vi "Humidification.vi"(10 "Humidifier":string="med", 11 "Controller in":refnum<class "Controller.lvclass">) -> ()   [LabVIEW 2018, in "Controller.lvlib" / "Controller.lvclass"]
doc: "This VI handles the humidifier loop."
uses:
  Controller.lvclass
  <vilib>/ActorFramework/Message Enqueuer/Message Enqueuer.lvclass
  Controls/eMap.ctl
  Devices/Vaisala Probe/Data/Vaisala Data.lvclass
  reusable/Session APIs/Session Log/System Log.lvclass
  <vilib>/ActorFramework/Actor/Actor.lvclass
  <vilib>/Platform/TimedLoop/XDataNode/XDataNode.xnode
  <vilib>/Platform/TimedLoop/XDataNode/nitl_modes.ctl
  <vilib>/Platform/TimedLoop/XDataNode/XDNodeRunTimeDep.lvlib
  <vilib>/Platform/TimedLoop/XDataNode/wakeup.ctl
  <vilib>/Platform/TimedLoop/XDataNode/timing_clust.ctl
  Devices/Meerstetter TEC/Data/mTEC Data.lvclass
  Devices/Alicat/Session Based/Data/Alicat Data.lvclass
  Update Controller Data MSG.lvclass
  Messages/Update Device Setpoint MSG/Update Device Setpoint.lvclass
  Data/humidity/humData.lvclass
  C:/Users/Labview/Documents/exscalabar_server/reusable/Data/Data.lvclass
  C:/Users/Labview/Documents/exscalabar_server/reusable/DAQ Device/Device/Generic Data Update Data MSG/Generic Update Data Message.lvclass
  C:/Program Files (x86)/National Instruments/LabVIEW 2018/vi.lib/ActorFramework/Message/Message.lvclass
  C:/Users/Labview/Documents/exscalabar_server/SuperActor/SuperActor.lvclass
  C:/Program Files (x86)/National Instruments/LabVIEW 2018/vi.lib/ActorFramework/Actor/Actor.lvclass
panel:
  out "TdReq":dbl
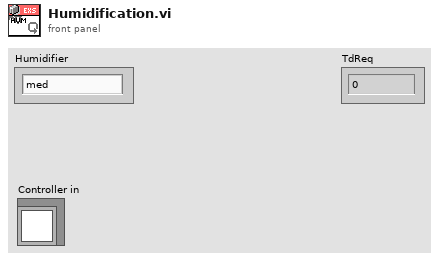
[diagram p1: front panel]
types:
  T1 = typedef "Session - Root.lvclass/Session Handle.ctl" = refnum<data-value>
  T2 = typedef "XDNodeRunTimeDep.lvlib/timing_clust.ctl" = cluster{"Expected End [f-1]":u64, "Actual End [f-1]":u64, "Finished Late? [f-1]":bool, "Expected End [i-1]":u64, "Actual End [i-1]":u64, "Finished Late? [i-1]":bool, "Expected Start [i]":u64, "Actual Start [i]":u64, "Expected Start [f]":u64, "Actual Start [f]":u64, "Source Name":string, "Structure Name":string, "Period":i64, "Deadline":i64, "Offset":i64, "Start":i64, "Priority":i32, "Timeout":i32, "Mode":T3, "Wakeup Reason":T4, "Error":errorcluster, "Source Type":string, "Secondary Source Type":string, "Global End Time":u64, "Global Start Time":u64, "Frame Duration":u64, "Iteration Duration":u64, "Assigned CPU":i32, "I/O Scan Engine Mode":u32}
  T3 = typedef "XDNodeRunTimeDep.lvlib/nitl_modes.ctl" = enum32{"No Change", "Process missed periods, maintain original phase", "Discard missed periods, maintain original phase", "Process missed periods, ignore original phase", "Discard missed periods, ignore original phase"}
  T4 = typedef "XDNodeRunTimeDep.lvlib/wakeup.ctl" = enum32{"Normal", "Aborted", "Asynchronous wakeup", "Timing source error", "Timed loop error", "Timeout"}
  T5 = typedef "Controller.lvlib/Controller.lvclass/eMap.ctl" = cluster{"Enqueuer":refnum<class "Message Enqueuer.lvclass">, "Active":bool}
  T6 = cluster{"Heff":dbl, "Leff":dbl, "dt":dbl, "smooth":dbl, "RHsp":dbl}
  T7 = cluster{"P":sgl, "T":sgl, "Q":sgl, "Qsp":sgl, "Q0":sgl}
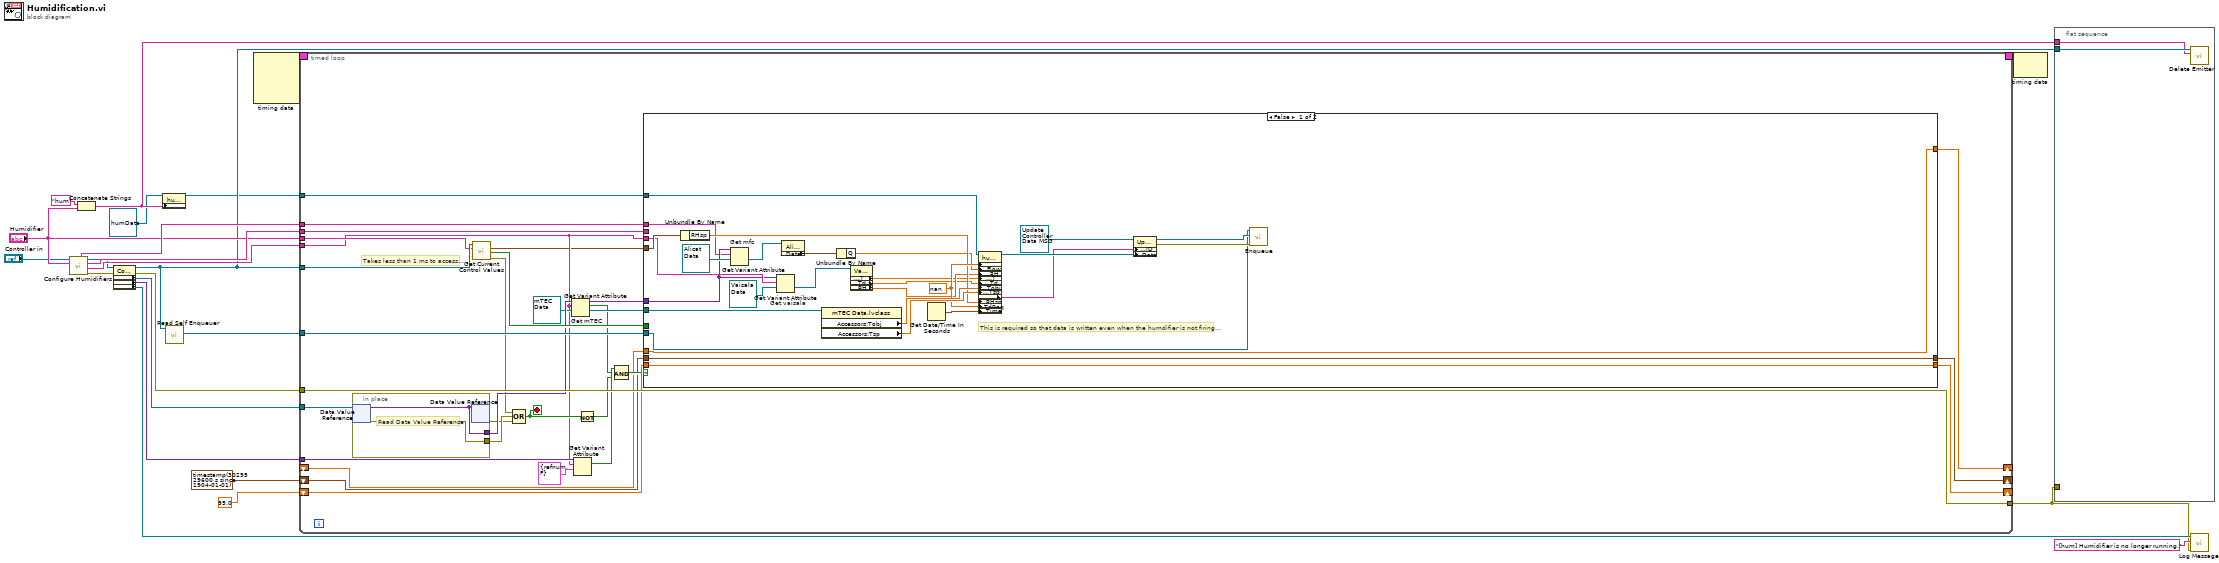
[diagram p0: block diagram]
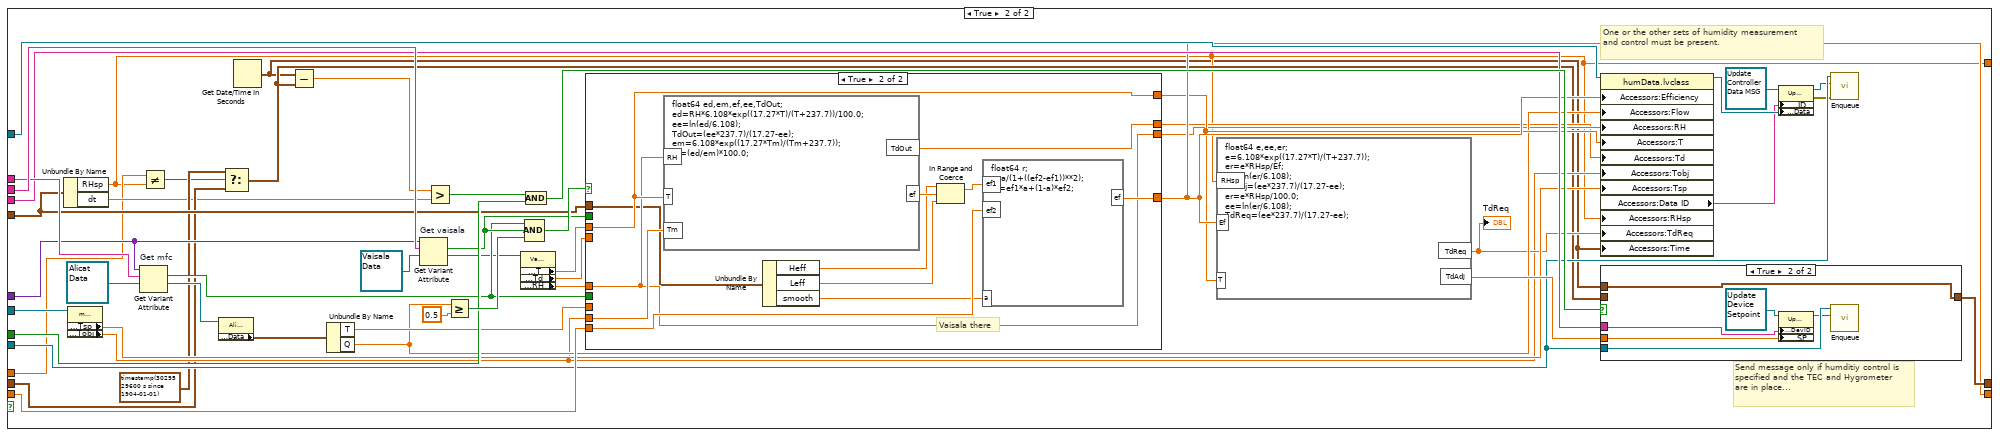
[diagram p2: hidden frame]
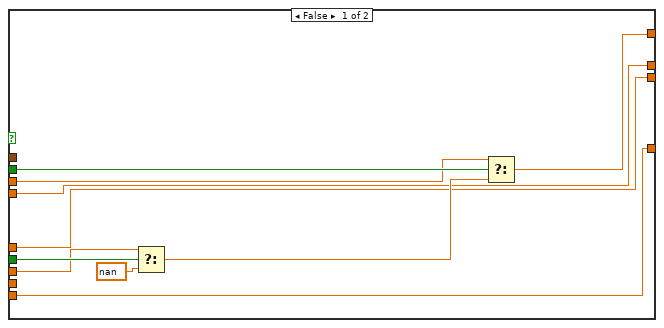
[diagram p3: hidden frame]
diagram:
  n1 = call "Configure Humidifiers.vi"("Humidifier"="Humidifier", "Controller in"="Controller in") -> ("error out"=w19:errorcluster, "TEC Handle"=w23:string, "Vaisala Handle"=w22:string, "Controller Out"=w20:refnum<class "Controller.lvclass">, "MFC"=w12:string)  [unwired: 5 in]
  n2 = Concatenate Strings("hum" ("Data ID"), "Humidifier") -> (w4:string)
  n3 = property class="Controller"(reference=w20, error in=w19) -> (reference out=w7:refnum<class "Controller.lvclass">, error out=w18:errorcluster, "Accessors:Data Map"=w8:refnum<data-value>, "Accessors:Enqueuer Map"=w21:variant, "Accessors:Log Session"=w17:T1)
  n4 = property class="humData.lvclass"(reference=refnum<class "humData.lvclass"> refnum ("humData.lvclass"), "Accessors:Data ID"=w4) -> (reference out=w3:refnum<class "humData.lvclass">)  [unwired: 1 in, 1 out]
  n5 = call <vilib>:"Read Self Enqueuer.vi"("Actor"=w7) -> ("Self Enqueuer"=w5:refnum<class "Message Enqueuer.lvclass">)  [unwired: 10 in]
  n6 = node-c288() -> (w14:T2)  [unwired: 4 in]
  n7 = timed-loop {
    tunnel: w23 -> [w29]
    tunnel: w22 -> [w54]
    tunnel: w21 -> [w49]
    tunnel: w8 -> [w42]
    tunnel: w7 -> [w52]
    tunnel: w18 -> [w50]
    tunnel: [w50] -> w6
    tunnel: w3 -> [w24]
    tunnel: w5 -> [w53]
    tunnel: "Humidifier" -> [w51]
    timing: w14 -> [_]
    timing-out: [_] -> w13
    tunnel: w12 -> [w48]
    shift-right: [w43] -> _
    shift-left: 95.0 -> [w47]
    shift-right: [w46] -> _
    shift-left: timestamp(3029529600 s since 1904-01-01) -> [w26]
    shift-right: [w28] -> _
    shift-left: _ -> [w25]
    stop <- w32 stop-if-true
    # "Takes less than 1 ms to access..."
    n8 = in-place {
      in-place-border: [w164] -> w40
      in-place-border: [w163] -> w34
      # "Read Data Value Reference"
      n9 = in-place-dvr #1(w42) -> (w164:variant, w163:errorcluster)
      n10 = in-place-dvr #1(w164) -> (w33:errorcluster)  [unwired: 1 out]
    }
    n11 = call "Get Current Control Values.vi"("Humidifier"=w51, "Controller in"=w52) -> ("error out"=w30:errorcluster, "Ctl"=w44:bool, "Control values"=w27:T6)  [unwired: 6 in, 1 out]
    n12 = Compound Arithmetic op=OR(w30, w34, w33) -> (w32:bool)
    n13 = Get Variant Attribute "Get mTEC"(Variant=w40, name=w29, default value (empty Variant)=refnum<class "mTEC Data.lvclass"> refnum ("Meerstetter Lib.lvlib:mTEC Data.lvclass")) -> (duplicate Variant=w39:variant, found=w37:bool, value=w41:refnum<class "mTEC Data.lvclass">)  [unwired: 1 in, 1 out]
    n14 = Get Variant Attribute(Variant=w49, name=w29, default value (empty Variant)=T5 {"Enqueuer"=refnum, "Active"=FALSE} ("eMap")) -> (found=w38:bool)  [unwired: 1 in, 3 out]
    n15 = Not(x=w32) -> (.not. x?=w31:bool)
    n16 = Compound Arithmetic op=AND(w38, w37, w31) -> (w36:bool)
    n17 = case shown="False" w36 {
      tunnel: w54 -> [_ w133]
      tunnel: w24 -> [w76 w107]
      tunnel: w53 -> [w75 w110]
      tunnel: w48 -> [w58 w132]
      tunnel: w47 -> [w82 w131]
      tunnel: [w83 w130] -> w46
      tunnel: w26 -> [w83 w89]
      tunnel: w44 -> [_ w119]
      tunnel: [w82 w105] -> w43
      tunnel: w41 -> [w74 w116]
      tunnel: w39 -> [w59 w122]
      tunnel: w29 -> [w65 w111]
      tunnel: [w67 w85] -> w28
      tunnel: w27 -> [w70 w92]
      tunnel: w25 -> [w67 w86]
      frame False {
        w71 = sgl nan ("Data")
        # "This is required so that data is written even when the humdifier is not firing..."
        n18 = Unbundle By Name(w70) -> ("RHsp"=w69:dbl)
        n19 = Get Variant Attribute "Get mfc"(Variant=w59, name=w58, default value (empty Variant)=refnum<class "Alicat Data.lvclass"> refnum ("Alicat Lib.lvlib:Alicat Data")) -> (value=w57:refnum<class "Alicat Data.lvclass">)  [unwired: 1 in, 3 out]
        n20 = Get Variant Attribute "Get vaisala"(Variant=w59, name=w65, default value (empty Variant)=refnum<class "Vaisala Data.lvclass"> refnum ("Vaisala Library.lvlib:Vaisala Data")) -> (value=w64:refnum<class "Vaisala Data.lvclass">)  [unwired: 1 in, 3 out]
        n21 = property class="Alicat Data"(reference=w57) -> ("Accessors:Data"=w56:T7)  [unwired: 1 in, 2 out]
        n22 = property class="mTEC Data.lvclass"(reference=w74) -> ("Accessors:Tobj"=w72:dbl, "Accessors:Tsp"=w73:dbl)  [unwired: 1 in, 2 out]
        n23 = Unbundle By Name(w56) -> ("Q"=w55:sgl)
        n24 = property class="Vaisala Data"(reference=w64) -> ("Accessors:T"=w62:dbl, "Accessors:Td"=w61:dbl, "Accessors:RH"=w63:dbl)  [unwired: 1 in, 2 out]
        n25 = Get Date/Time In Seconds() -> (seconds since 1Jan1904=w68:timestamp)
        n26 = property class="humData.lvclass"(reference=w76, "Accessors:Efficiency"=w71, "Accessors:Flow"=w55, "Accessors:RH"=w63, "Accessors:T"=w62, "Accessors:Td"=w61, "Accessors:Tobj"=w72, "Accessors:Tsp"=w73, "Accessors:RHsp"=w69, "Accessors:TdReq"=w71, "Accessors:Time"=w68) -> (reference out=w81:refnum<class "humData.lvclass">, "Accessors:Data ID"=w77:string)  [unwired: 1 in, 1 out]
        n27 = property class="Update Data MSG"(reference=refnum<class "Update Controller Data MSG.lvclass"> refnum ("Controller:Update Data MSG"), "Accessors:ID"=w77, "Accessors:Data"=w81) -> (reference out=w79:refnum<class "Update Controller Data MSG.lvclass">, error out=w80:errorcluster)  [unwired: 1 in]
        n28 = call <vilib>:"Enqueue.vi"("error in (no error)"=w80, "Message"=w79, "Message Enqueuer in"=w75) -> ()  [unwired: 7 in, 2 out]
      }
      frame True {
        # "Send message only if humditiy control is specified and the TEC and Hygrometer are in place..."
        # "One or the other sets of humidity measurement and control must be present."
        n29 = Unbundle By Name(w92) -> ("RHsp"=w85:dbl, "dt"=w87:dbl)
        n30 = property class="mTEC Data.lvclass"(reference=w116) -> ("Accessors:Tsp"=w100:dbl, "Accessors:Tobj"=w93:dbl)  [unwired: 1 in, 2 out]
        n31 = Get Variant Attribute "Get mfc"(Variant=w122, name=w132, default value (empty Variant)=refnum<class "Alicat Data.lvclass"> refnum ("Alicat Lib.lvlib:Alicat Data")) -> (found=w112:bool, value=w117:refnum<class "Alicat Data.lvclass">)  [unwired: 1 in, 2 out]
        n32 = Not Equal?(x=w86, y=w85) -> (x != y?=w90:bool)
        n33 = property class="Alicat Data"(reference=w117) -> ("Accessors:Data"=w126:T7)  [unwired: 1 in, 2 out]
        n34 = Select(t=timestamp(3029529600 s since 1904-01-01), s=w90, f=w89) -> (s? t:f=w88:timestamp)
        n35 = Get Date/Time In Seconds() -> (seconds since 1Jan1904=w84:timestamp)
        n36 = Subtract(x=w84, y=w88) -> (x-y=w129:dbl)
        n37 = Unbundle By Name(w126) -> ("T"=w113:sgl, "Q"=w102:sgl)
        n38 = Get Variant Attribute "Get vaisala"(Variant=w122, name=w133, default value (empty Variant)=refnum<class "Vaisala Data.lvclass"> refnum ("Vaisala Library.lvlib:Vaisala Data")) -> (found=w114:bool, value=w98:refnum<class "Vaisala Data.lvclass">)  [unwired: 1 in, 2 out]
        n39 = Greater?(x=w129, y=w87) -> (0:w121:bool)
        n40 = Greater Or Equal?(x=w102, y=sgl 0.5) -> (x >= y?=w123:bool)
        n41 = property class="Vaisala Data"(reference=w98) -> ("Accessors:T"=w97:dbl, "Accessors:Td"=w96:dbl, "Accessors:RH"=w95:dbl)  [unwired: 1 in, 2 out]
        n42 = And(x=w121, y=w119) -> (x .and. y?=w120:bool)
        n43 = Compound Arithmetic op=AND(w112, w114, w123) -> (w124:bool)
        n44 = case shown="True" w124 {
          tunnel: [w142 w150] -> w103
          tunnel: w93 -> [_ w155]
          tunnel: w131 -> [w139 w153]
          tunnel: w113 -> [w134 _]
          tunnel: w114 -> [w143 _]
          tunnel: w112 -> [w140 _]
          tunnel: [w139 w154] -> w105
          tunnel: [w135 w149] -> w101
          tunnel: [w136 w148] -> w99
          tunnel: w97 -> [w137 w150]
          tunnel: w96 -> [w136 _]
          tunnel: w95 -> [w135 w149]
          tunnel: w92 -> [_ w147]
          frame False {
            n45 = Select(t=w134, s=w140, f=sgl nan) -> (s? t:f=w141:sgl)
            n46 = Select(t=w137, s=w143, f=w141) -> (s? t:f=w142:dbl)
          }
          frame True {
            # "Vaisala there"
            n47 = formula code="float64 ed,em,ef,ee,TdOut;\ned=RH*6.108*exp((17.27*T)/(T+237.7))/100.0;\nee=ln(ed/6.108);\nTdOut=(ee*237.7)/(17.27-ee);\nem=6.108*exp((17.27*Tm)/(Tm+237.7));\nef=(ed/em)*100.0;"("T"=w150, "Tm"=w155, "RH"=w149) -> ("ef"=w152:dbl, "TdOut"=w148:dbl)
            n48 = Unbundle By Name(w147) -> ("Heff"=w146:dbl, "Leff"=w145:dbl, "smooth"=w144:dbl)
            n49 = In Range and Coerce(upper limit=w146, x=w152, lower limit=w145) -> (coerced(x)=w151:dbl)  [unwired: 1 out]
            n50 = formula code="float64 r;\nr=a/(1+((ef2-ef1))**2);\nef=ef1*a+(1-a)*ef2;"("ef1"=w151, "ef2"=w153, "a"=w144) -> ("ef"=w154:dbl)
          }
        }
        n51 = formula code="float64 e,ee,er;\ne=6.108*exp((17.27*T)/(T+237.7));\ner=e*RHsp/Ef;\nee=ln(er/6.108);\nTdAdj=(ee*237.7)/(17.27-ee);\ner=e*RHsp/100.0;\nee=ln(er/6.108);\nTdReq=(ee*237.7)/(17.27-ee);"("RHsp"=w85, "Ef"=w105, "T"=w103) -> ("TdReq"=w94:dbl, "TdAdj"=w128:dbl)
        "TdReq" <- w94
        n52 = property class="humData.lvclass"(reference=w107, "Accessors:Efficiency"=w105, "Accessors:Flow"=w102, "Accessors:RH"=w101, "Accessors:T"=w103, "Accessors:Td"=w99, "Accessors:Tobj"=w93, "Accessors:Tsp"=w100, "Accessors:RHsp"=w85, "Accessors:TdReq"=w94, "Accessors:Time"=w84) -> (reference out=w106:refnum<class "humData.lvclass">, "Accessors:Data ID"=w104:string)  [unwired: 1 in, 1 out]
        n53 = case shown="True" w120 {
          tunnel: w128 -> [_ w162]
          tunnel: w88 -> [w156 _]
          tunnel: w84 -> [_ w161]
          tunnel: [w156 w161] -> w130
          tunnel: w111 -> [_ w160]
          tunnel: w110 -> [_ w159]
          frame False {
          }
          frame True {
            n54 = property class="Update Device Setpoint"(reference=refnum<class "Update Device Setpoint.lvclass"> refnum ("Controller.lvlib:Update Device Setpoint"), "Accessors:DevID"=w160, "Accessors:SP"=w162) -> (reference out=w157:refnum<class "Update Device Setpoint.lvclass">)  [unwired: 1 in, 1 out]
            n55 = call <vilib>:"Enqueue.vi"("Message"=w157, "Message Enqueuer in"=w159) -> ()  [unwired: 8 in, 2 out]
          }
        }
        n56 = property class="Update Data MSG"(reference=refnum<class "Update Controller Data MSG.lvclass"> refnum ("Controller:Update Data MSG"), "Accessors:ID"=w104, "Accessors:Data"=w106) -> (reference out=w109:refnum<class "Update Controller Data MSG.lvclass">, error out=w108:errorcluster)  [unwired: 1 in]
        n57 = call <vilib>:"Enqueue.vi"("error in (no error)"=w108, "Message"=w109, "Message Enqueuer in"=w110) -> ()  [unwired: 7 in, 2 out]
      }
    }
  }
  n58 = node-c288(w13) -> ()  [unwired: 1 out]
  n59 = flat-sequence {
    tunnel: w7 -> [w168]
    tunnel: w6 -> [_]
    tunnel: w4 -> [w167]
    frame #0 {
      n60 = call "Delete Emitter.vi"("Emitter"=w167, "Controller in"=w168) -> ()  [unwired: 8 in, 2 out]
    }
  }
  n61 = call "Log Message.vi"("error in"=w6, "MSG In"="[hum] Humidifier is no longer running.", "session in"=w17) -> ()  [unwired: 7 in, 2 out]
